vi "Remove Nan & optionally 0 from SGL array.vi"(4 "Remove zeros? (T)":bool=TRUE, 5 "array in":sgl[](array[numeric])=[35.0, nan, 0.0]) -> (2 "arrayout":sgl[](array[numeric])=[35.0])   [LabVIEW 2010]
doc: "Removes Nan & zereo from input array and returns."
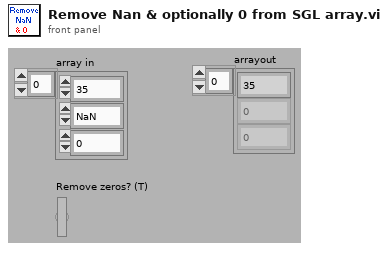
[diagram p1: front panel]
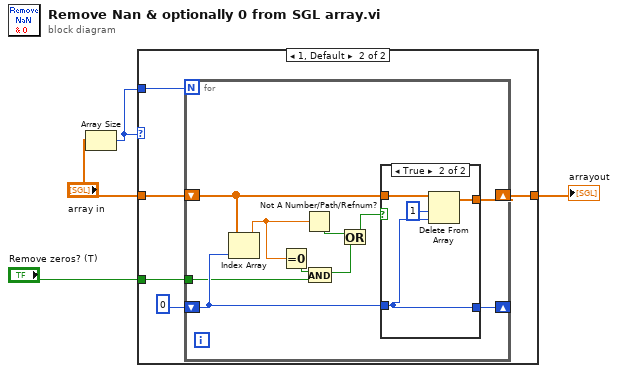
[diagram p0: block diagram]
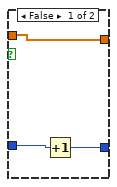
[diagram p3: hidden frame]
diagram:
  n1 = Array Size(array="array in") -> (size(s)=w2:i32)
  n2 = case shown="1, Default" w2 {
    tunnel: "array in" -> [w5 w10]
    tunnel: w2 -> [_ w9]
    tunnel: [w5 w8] -> w3
    tunnel: "Remove zeros? (T)" -> [_ w6]
    frame 0 {
    }
    frame 1, Default {
      n3 = for {
        N: w9 -> [_]
        shift-right: [w19] -> w8
        shift-left: w10 -> [w20]
        shift-right: [w17] -> _
        shift-left: 0 -> [w18]
        tunnel: w6 -> [w12]
        n4 = Index Array(array=w20, index=w18) -> (element=w15:sgl)
        n5 = Equal To 0?(x=w15) -> (x = 0?=w13:bool)
        n6 = Not A Number/Path/Refnum?(number/path/refnum=w15) -> (NaN/Path/Refnum?=w16:bool)
        n7 = And(x=w13, y=w12) -> (x .and. y?=w11:bool)
        n8 = Or(x=w16, y=w11) -> (x .or. y?=w14:bool)
        n9 = case shown="True" w14 {
          tunnel: w20 -> [w23 w27]
          tunnel: [w23 w25] -> w19
          tunnel: w18 -> [w22 w24]
          tunnel: [w21 w24] -> w17
          frame False {
            n10 = Increment(x=w22) -> (x+1=w21:i32)
          }
          frame True {
            n11 = Delete From Array(array=w27, length=1, index=w24) -> (array with subset deleted=w25:sgl[])  [unwired: 1 out]
          }
        }
      }
    }
  }
  "arrayout" <- w3
